vi "Split.vi"(6 "Groups":string[][](array[string]), 8 "error in (no error)":errorcluster caption="entrée d'erreur (pas d'erreur)", 9 "y":string[][](array[string]), 10 "X":string[][](array[string]), 11 "GroupKFold.lvclass":refnum<class "GroupKFold.lvclass">) -> (0 "error out":errorcluster caption="sortie d'erreur", 2 "Split":T1(array[cluster]), 3 "GroupKFold.lvclass":refnum<class "GroupKFold.lvclass">)   [LabVIEW 2020, in "GroupKFold.lvclass"]
doc: "Return : \n- train : ndarray\n The training set indices for that split.\n\n- test : ndarray\n The testing set indices for that split."
uses:
  GroupKFold.lvclass
  GroupKFold.lvclass/GroupKFold.ctl
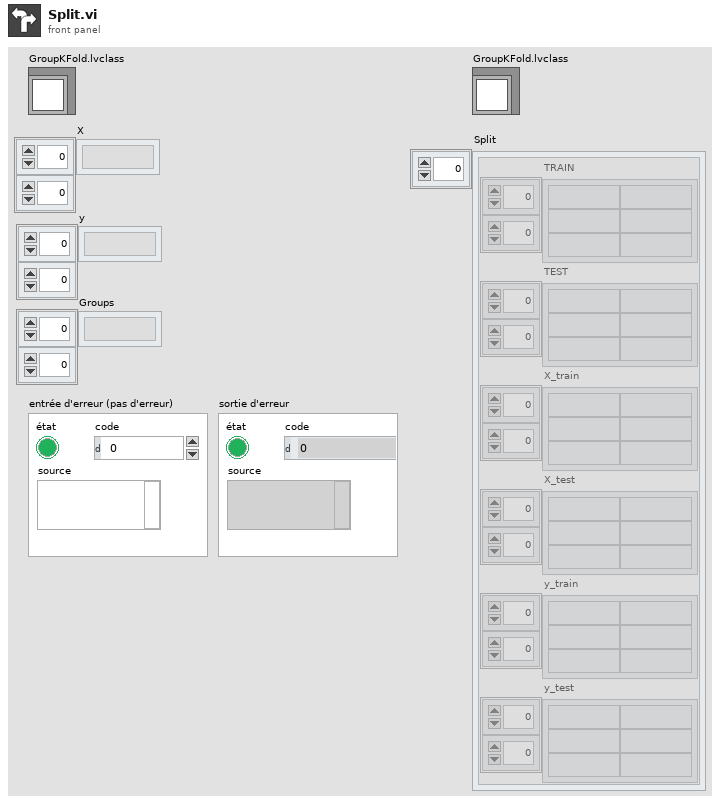
[diagram p1: front panel]
types:
  T1 = cluster{"TRAIN":string[][], "TEST":string[][], "X_train":string[][], "X_test":string[][], "y_train":string[][], "y_test":string[][]}[]
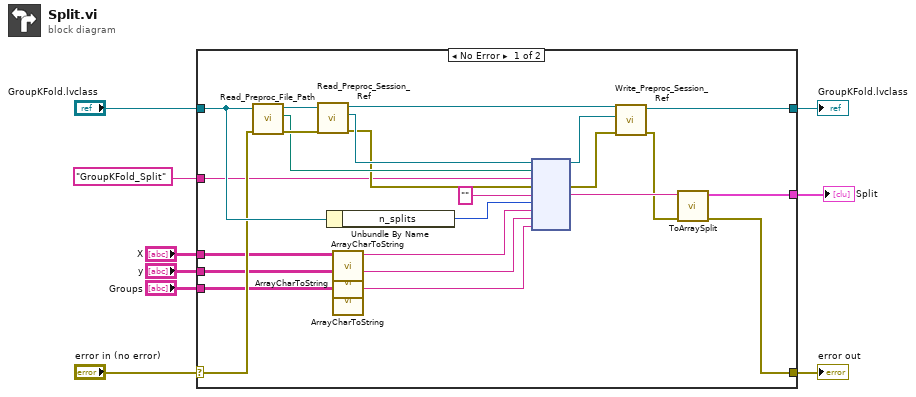
[diagram p0: block diagram]
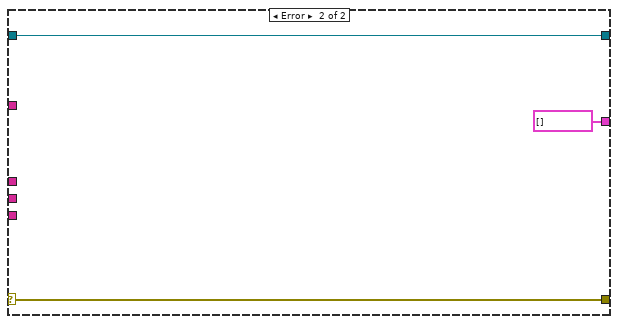
[diagram p2: hidden frame]
diagram:
  n1 = case shown="No Error" "error in (no error)" {
    selector: "error in (no error)" -> [w23 w36]
    tunnel: [w11 w36] -> w8
    tunnel: [w20 w35] -> w6
    tunnel: "GroupKFold.lvclass" -> [w24 w35]
    tunnel: "GroupKFold_Split" -> [w22 _]
    tunnel: "X" -> [w19 _]
    tunnel: "y" -> [w18 _]
    tunnel: "Groups" -> [w17 _]
    tunnel: [w10 T1 [] ("Split")] -> w1
    frame No Error {
      n2 = call-dynamic "Read_Preproc_File_Path.vi"("error in (no error)"=w23, "Python in"=w24) -> ("error out"=w32:errorcluster, "File_Path"=w31:path, "Python out"=w33:refnum<class "GroupKFold.lvclass">)  [unwired: 7 in]
      n3 = call-dynamic "Read_Preproc_Session_Ref.vi"("error in (no error)"=w32, "Python in"=w33) -> ("error out"=w29:errorcluster, "Session_ref"=w30:refnum<k35>, "Python out"=w28:refnum<class "GroupKFold.lvclass">)  [unwired: 7 in]
      n4 = Unbundle By Name(w24) -> ("n_splits"=w21:i32)
      n5 = call "ArrayCharToString.vi"("TAB"=w19) -> ("Instruction"=w16:string)  [unwired: 10 in]
      n6 = call "ArrayCharToString.vi"("TAB"=w18) -> ("Instruction"=w15:string)  [unwired: 10 in]
      n7 = call "ArrayCharToString.vi"("TAB"=w17) -> ("Instruction"=w14:string)  [unwired: 10 in]
      n8 = node(w30, w31, w22, w29, "", w21, w16, w15, w14) -> (w26:refnum<k35>, w27:errorcluster, w13:string)  [unwired: 4 in, 2 out]
      n9 = call-dynamic "Write_Preproc_Session_Ref.vi"("error in (no error)"=w27, "Session_ref"=w26, "Python in"=w28) -> ("error out"=w12:errorcluster, "Python out"=w20:refnum<class "GroupKFold.lvclass">)  [unwired: 7 in]
      n10 = call "ToArraySplit.vi"("sortie d'erreur"=w12, "Return value"=w13) -> ("sortie d'erreur"=w11:errorcluster, "Split"=w10:T1)  [unwired: 8 in]
    }
    frame Error {
    }
  }
  "error out" <- w8
  "GroupKFold.lvclass" <- w6
  "Split" <- w1
